vi "set_device_state.vi"(8 "error in":errorcluster, 10 "state_in":T1, 11 "TCP Network Connection in":refnum<k5>) -> (0 "error out":errorcluster, 2 "error?":bool, 3 "TCP Network Connection out":refnum<k5>)   [LabVIEW 2021]
uses:
  typedefs/general_states.ctl
  typedefs/w5500_cmd.ctl
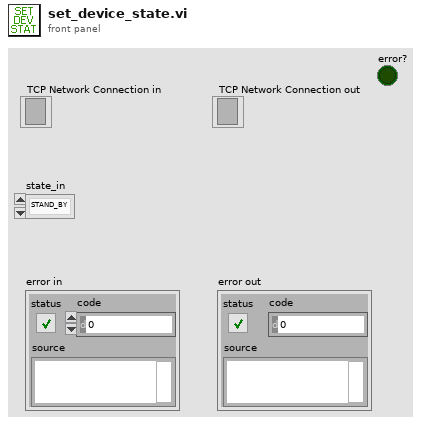
[diagram p1: front panel]
types:
  T1 = typedef "general_states.ctl" = enum16{"STAND_BY", "IDLE", "WAIT_TRIG", "RECORD", "DATA_RDY", "ERROR"}
  T2 = typedef "w5500_cmd.ctl" = enum32{"LAN_TRANS_START", "LAN_DATA_SZ", "LAN_CHUNK_SEND", "LAN_CHUNK_ACK", "LAN_DEVS_INFO", "LAN_DEVS_NUM", "LAN_DEVS_EXS", "LAN_DEVS_ACK", "LAN_CMD_ACK", "LAN_CMD_FIN", "LAN_SND_STAT", "LAN_REQ_STAT", "LAN_ANS_STAT", "LAN_ERR_STAT", "LAN_SETT_SET", "LAN_SETT_GET", "LAN_SETT_ACK", "LAN_SETT_ERR"}
  T3 = typedef "w5500_pck.ctl" = cluster{"cmd_type":T2, "pck_num":u32, "dev_id":u32, "data":u8[]}
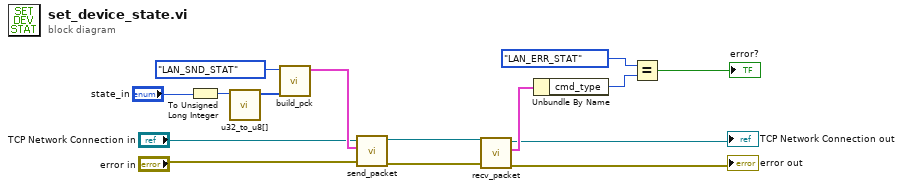
[diagram p0: block diagram]
diagram:
  n1 = To Unsigned Long Integer(number="state_in") -> (unsigned 32bit integer=w13:u32)
  n2 = call "u32_to_u8[].vi"("data_in"=w13) -> ("arr_out"=w14:u8[])  [unwired: 10 in]
  n3 = call "build_pck.vi"("data in"=w14, "cmd_type"=w5500_cmd."LAN_SND_STAT") -> ("w5500_pck"=w11:T3)  [unwired: 9 in]
  n4 = call "send_packet.vi"("error in (no error)"="error in", "w5500_pck in"=w11, "TCP Network Connection in"="TCP Network Connection in") -> ("error out"=w4:errorcluster, "TCP Network Connection out"=w5:refnum<k5>)  [unwired: 7 in]
  n5 = call "recv_packet.vi"("error in (no error)"=w4, "TCP Network Connection in"=w5) -> ("error out"=→"error out":errorcluster, "w5500_pck"=w6:T3, "TCP Network Connection out"=→"TCP Network Connection out":refnum<k5>)  [unwired: 7 in]
  n6 = Unbundle By Name(w6) -> ("cmd_type"=w7:T2)
  n7 = Equal?(x=w5500_cmd."LAN_ERR_STAT" ("cmd_type"), y=w7) -> (x = y?=→"error?":bool)
